vi "MTMount_getSample_MirrorCover.vi"(8 "error in (no error)":errorcluster, 11 "Mirror_Cover_Ctl":T1) -> (0 "error out":errorcluster, 2 "function return":i32, 3 "Mirror_Cover_Ctl out":T1)   [LabVIEW 2018, in "SALLV_MTMount.lvlib"]
doc: "int MTMount_shm_getSample_Mirror_CoverLV(MTMount_Mirror_CoverLV *Mirror_Cover_Ctl );"
uses:
  SALLV_MTMount.lvlib
  DataTypes/Mirror_Cover.ctl
  SALLV_MTMount.so
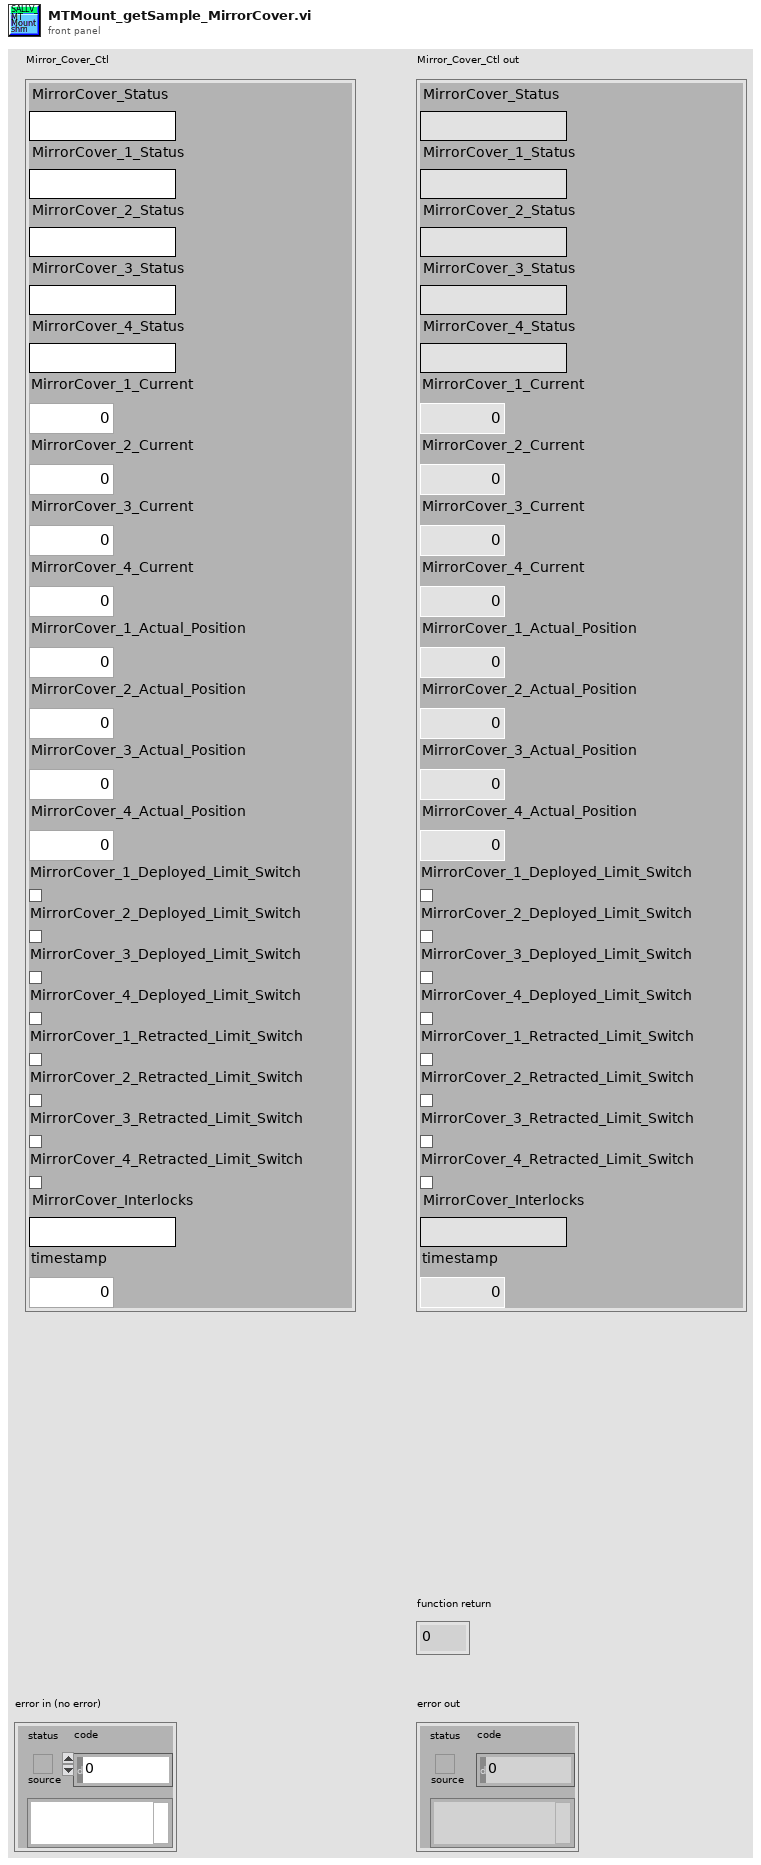
[diagram p1: front panel]
types:
  T1 = typedef "SALLV_MTMount.lvlib/Mirror_Cover.ctl" = cluster{"MirrorCover_Status":string, "MirrorCover_1_Status":string, "MirrorCover_2_Status":string, "MirrorCover_3_Status":string, "MirrorCover_4_Status":string, "MirrorCover_1_Current":dbl, "MirrorCover_2_Current":dbl, "MirrorCover_3_Current":dbl, "MirrorCover_4_Current":dbl, "MirrorCover_1_Actual_Position":dbl, "MirrorCover_2_Actual_Position":dbl, "MirrorCover_3_Actual_Position":dbl, "MirrorCover_4_Actual_Position":dbl, "MirrorCover_1_Deployed_Limit_Switch":bool, "MirrorCover_2_Deployed_Limit_Switch":bool, "MirrorCover_3_Deployed_Limit_Switch":bool, "MirrorCover_4_Deployed_Limit_Switch":bool, "MirrorCover_1_Retracted_Limit_Switch":bool, "MirrorCover_2_Retracted_Limit_Switch":bool, "MirrorCover_3_Retracted_Limit_Switch":bool, "MirrorCover_4_Retracted_Limit_Switch":bool, "MirrorCover_Interlocks":string, "timestamp":dbl}
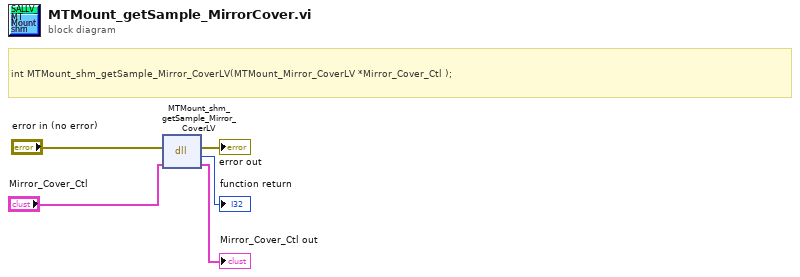
[diagram p0: block diagram]
diagram:
  # "int MTMount_shm_getSample_Mirror_CoverLV(MTMount_Mirror_CoverLV *Mirror_Cover_Ctl );"
  n1 = dll-call lib="home/ttsai/Document/salApiMTMount/SALLV_MTMount/SALLV_MTMount.*" fn="MTMount_shm_getSample_Mirror_CoverLV"(error in="error in (no error)", "Mirror_Cover_Ctl"="Mirror_Cover_Ctl") -> (error out=→"error out":errorcluster, →"function return":i32, "Mirror_Cover_Ctl"=→"Mirror_Cover_Ctl out":T1)  [unwired: 2 in, 1 out]
